vi "View.vi"(4 "dt":dbl=0.0001 format="%#_13g", 5 "Data type":T1 items=["AXON", "HEKA"], 6 "Event #":i16=4, 7 "Sweep #":i16=4, 8 "Baseline info new OUT":cluster{dbl[][]}[](array[cluster]), 9 "Sweep trace (2D) In":cluster{"Ramp Pattern":dbl[], "X":dbl[]}[][](array[cluster]), 10 "Detected Event (1D) In":cluster{dbl[][]}[](array[cluster])) -> (0 "event":cluster{dbl[], dbl[]}[](graph), 2 "Y range":T2, 3 "출력 클러스터":T3)   [LabVIEW 2017]
uses:
  Data type_new.ctl
  <vilib>/Analysis/baseanly.llb/Mean (DBL).vi
  <vilib>/Analysis/NI_AALPro.lvlib
  <vilib>/Analysis/NI_AALBase.lvlib
panel:
  out "Mean baseline (pA)":dbl
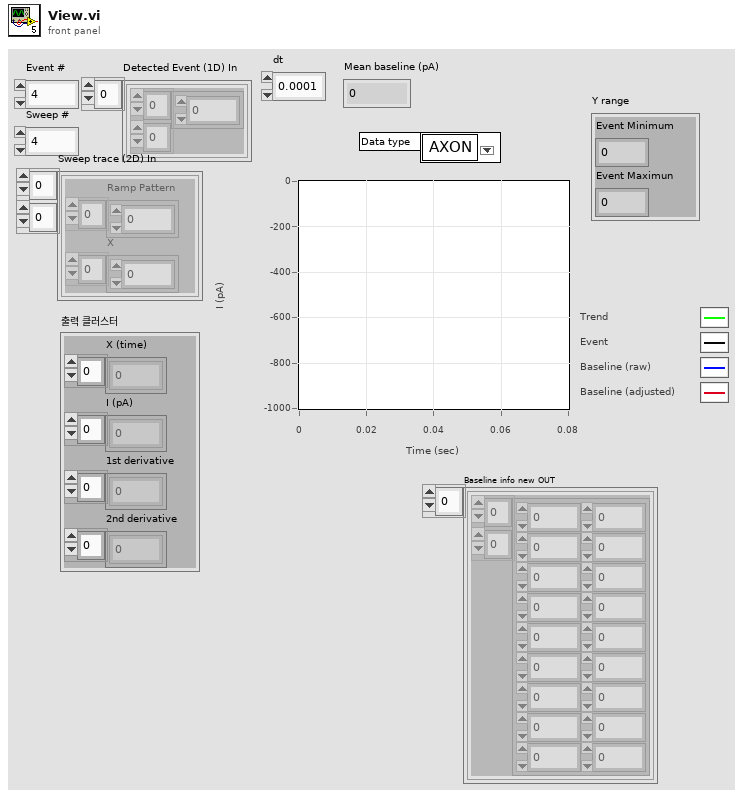
[diagram p1: front panel]
types:
  T1 = typedef "Data type_new.ctl" = u16
  T2 = cluster{"Event Minimum":dbl, "Event Maximun":dbl}
  T3 = cluster{"X (time)":dbl[], "I (pA)":dbl[], "1st derivative":dbl[], "2nd derivative":dbl[]}
  T4 = cluster{dbl[], dbl[], "dX/dt":dbl[], "dX/dt":dbl[]}
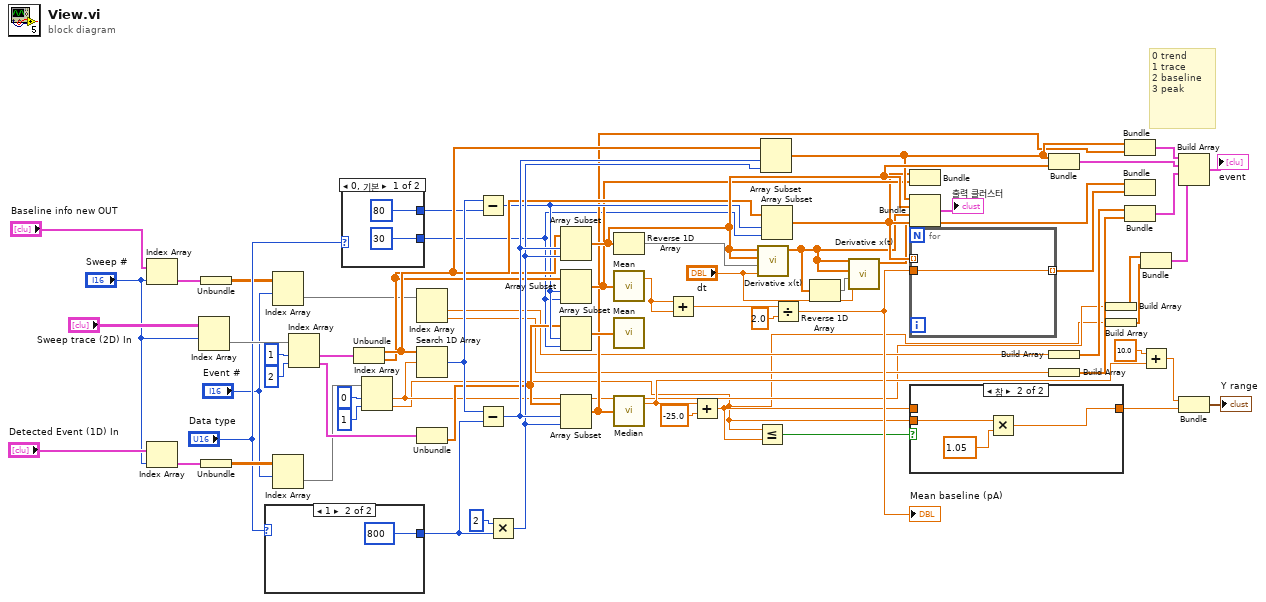
[diagram p0: block diagram]
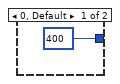
[diagram p2: hidden frame]
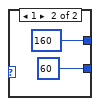
[diagram p3: hidden frame]
diagram:
  # "0 trend\n1 trace\n2 baseline\n3 peak"
  n1 = Index Array(array="Baseline info new OUT", index="Sweep #") -> (element=w21:cluster{dbl[][]})
  n2 = Index Array(array="Detected Event (1D) In", index="Sweep #") -> (element=w68:cluster{dbl[][]})
  n3 = Index Array(array="Sweep trace (2D) In", index (row)="Sweep #") -> (element=w65:cluster{"Ramp Pattern":dbl[], "X":dbl[]}[])  [unwired: 1 in]
  n4 = Unbundle(w21) -> (w20:dbl[][])
  n5 = Unbundle(w68) -> (w41:dbl[][])
  n6 = case shown="1" "Data type" {
    tunnel: [400 800] -> w62
    frame 0, Default {
    }
    frame 1 {
    }
  }
  n7 = Index Array(array=w20, index (row)="Event #") -> (element=w18:dbl[])  [unwired: 1 in]
  n8 = Index Array(array=w41, index (row)="Event #") -> (element=w42:dbl[])  [unwired: 1 in]
  n9 = Index Array(array=w65, index #1=1 ("인덱스"), index #2=2 ("인덱스")) -> (element #1=w63:cluster{"Ramp Pattern":dbl[], "X":dbl[]}, element #2=w56:cluster{"Ramp Pattern":dbl[], "X":dbl[]})
  n10 = case shown="0, 기본" "Data type" {
    tunnel: [80 ("y") 160 ("y")] -> w27
    tunnel: [30 ("길이") 60 ("길이")] -> w26
    frame 0, Default {
    }
    frame 1 {
    }
  }
  n11 = Unbundle(w63) -> ("Ramp Pattern"=w51:dbl[], "X"=w50:dbl[])
  n12 = Index Array(array=w42, index #1=0 ("인덱스"), index #2=1 ("인덱스")) -> (element #1=w9:dbl, element #2=w8:dbl)
  n13 = Index Array(array=w18) -> (element #1=w17:dbl, element #2=w16:dbl)  [unwired: 2 in]
  n14 = Search 1D Array(1D array=w51, element=w9) -> (index of element=w52:i32)  [unwired: 1 in]
  n15 = Unbundle(w56) -> ("X"=w38:dbl[])  [unwired: 1 out]
  n16 = Subtract(x=w52, y=w27) -> (x-y=w49:i32)
  n17 = Subtract(x=w52, y=w62) -> (x-y=w55:i32)
  n18 = Multiply(x=2, y=w62) -> (x*y=w54:i32)
  n19 = Array Subset(array=w50, index=w55, length=w54) -> (w59:dbl[])
  n20 = Array Subset(array=w50, index=w49, length=w26) -> (w48:dbl[])
  n21 = Array Subset(array=w38, index=w49, length=w26) -> (w47:dbl[])
  n22 = Array Subset(array=w38, index=w55, length=w54) -> (w37:dbl[])
  n23 = Reverse 1D Array(array=w59) -> (reversed array=w60:dbl[])
  n24 = call-poly <vilib>:"Mean.vi"("X"=w48) -> ("mean"=w25:dbl)  [unwired: 1 out]
  n25 = call-poly <vilib>:"Mean.vi"("X"=w47) -> ()  [unwired: 2 out]
  n26 = call <vilib>:"Median.vi"("X"=w37) -> ("median"=w35:dbl)  [unwired: 1 out]
  n27 = Add(x=w25, y=w25) -> (x+y=w46:dbl)
  n28 = Add(x=w35, y=-25.0) -> (x+y=w31:dbl)
  n29 = Less Or Equal?(x=w8, y=w31) -> (x <= y?=w32:bool)
  n30 = call <vilib>:"Derivative x(t).vi"("dt"="dt", "Final Condition"=w60, "Initial Condition"=w59, "X"=w59) -> ("dX/dt"=w4:dbl[])  [unwired: 6 in, 1 out]
  n31 = Array Subset(array=w51, index=w55, length=w54) -> (w53:dbl[])
  n32 = Array Subset(array=w51, index=w49, length=w26) -> (w44:dbl[])
  n33 = Divide(x=w46, y=2.0) -> (x/y=w39:dbl)
  "Mean baseline (pA)" <- w39
  n34 = Reverse 1D Array(array=w4) -> (reversed array=w3:dbl[])
  n35 = call <vilib>:"Derivative x(t).vi"("dt"="dt", "Final Condition"=w3, "Initial Condition"=w4, "X"=w4) -> ("dX/dt"=w1:dbl[])  [unwired: 6 in, 1 out]
  n36 = Bundle(w44, w48) -> ()  [unwired: 1 in, 1 out]
  n37 = Bundle(w53, w59, "dX/dt"=w4, "dX/dt"=w1) -> (→"출력 클러스터":T4)  [unwired: 1 in]
  n38 = for {
    tunnel: w44 -> [_] mode=indexing
    tunnel: [w75] -> w43 mode=indexing
    tunnel: w39 -> [w75]
  }
  n39 = case shown="참" w32 {
    tunnel: w8 -> [_ w79]
    tunnel: w31 -> [w76 _]
    tunnel: [w76 w77] -> w29
    frame False {
    }
    frame True {
      n40 = Multiply(x=w79, y=1.05) -> (x*y=w77:dbl)
    }
  }
  n41 = Bundle(w53, w59) -> (w12:cluster{dbl[], dbl[]})  [unwired: 1 in]
  n42 = Build Array(w17) -> (w15:dbl[])
  n43 = Build Array(w16) -> (w14:dbl[])
  n44 = Build Array(w9) -> (w7:dbl[])
  n45 = Build Array(w8) -> (w6:dbl[])
  n46 = Bundle(w53, w37) -> (w13:cluster{dbl[], dbl[]})  [unwired: 1 in]
  n47 = Bundle(w44, w43) -> ()  [unwired: 1 in, 1 out]
  n48 = Bundle(w15, w14) -> (w11:cluster{dbl[], dbl[]})  [unwired: 1 in]
  n49 = Bundle(w7, w6) -> (w5:cluster{dbl[], dbl[]})  [unwired: 1 in]
  n50 = Add(x=10.0, y=w35) -> (x+y=w30:dbl)
  n51 = Build Array(w13, w12, w11, w5) -> (→"event":cluster{dbl[], dbl[]}[])
  n52 = Bundle(w30, w29) -> (→"Y range":cluster{dbl, dbl})  [unwired: 1 in]
